vi "BH Druck  PACE Series Controller.vi"() -> ()   [LabVIEW 2022 SP3]
uses:
  <vilib>/Utility/error.llb/DialogType.ctl
  BH Druck PACE Series.lvclass
panel:
  out "Pressure":dbl format="%#.10g"
  out "+ve Source":dbl format="%#.10g"
  out "-ve Source":dbl format="%#.10g"
  in  "stop":bool
  out "Time to In Limits":string
  out "In Limits":bool
  out "Barometer":dbl format="%#.10g"
  in  "Enable Controller":bool
  in  "Slew Rate (0)":dbl
  in  "Slew Mode (Maximum)":string(combo)="max"
  in  "Overshoot (0: Not Allowed)":u16(ring)=1 items=["Not Allowed", "Allowed"]
  in  "Unit (mbar)":u16(ring) items=["mbar", "bar", "Pa", "hPa", "kPa", "mPa", "mmHg@0°C", "cmHg@0°C", "mHg@0°C", "inHg@0°C", "kg/cm2", "kg/m2", "mmH2O@4°C", "cmH2O@4°C", "mH2O@4°C", "mmH2O@20°C", "cmH2O@20°C", "mH2O@20°C", "torr", "atm", "psi", "lb/ft2", "inH2O@4°C", "inH2O@20°C", "inH2O@60°F", "ftH2O@4°C", "ftH2O@20°C", "ftH2O@60°F", "UserUnit1", "UserUnit2", "UserUnit3", "UserUnit4"]
  in  "Setpoint Value (0)":dbl
  out "Range":string
  out "-ve Full Scale":dbl
  out "+ve Full Scale":dbl
  in  "Channel (0: Channel A)":u16(ring) items=["Channel A", "Channel B"]
  in  "VISA resource name":refnum<visa-resource-name>
  # "(c)2010-2017 BH  Druck Ltd.  ALL RIGHTS RESERVED."
  # "Select port and channel"
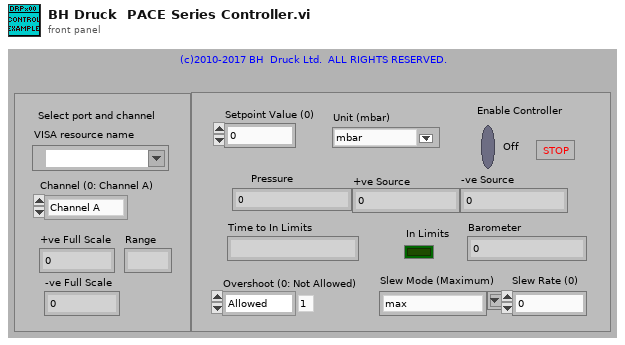
[diagram p1: front panel]
types:
  T1 = typedef "DialogType.ctl" = u16
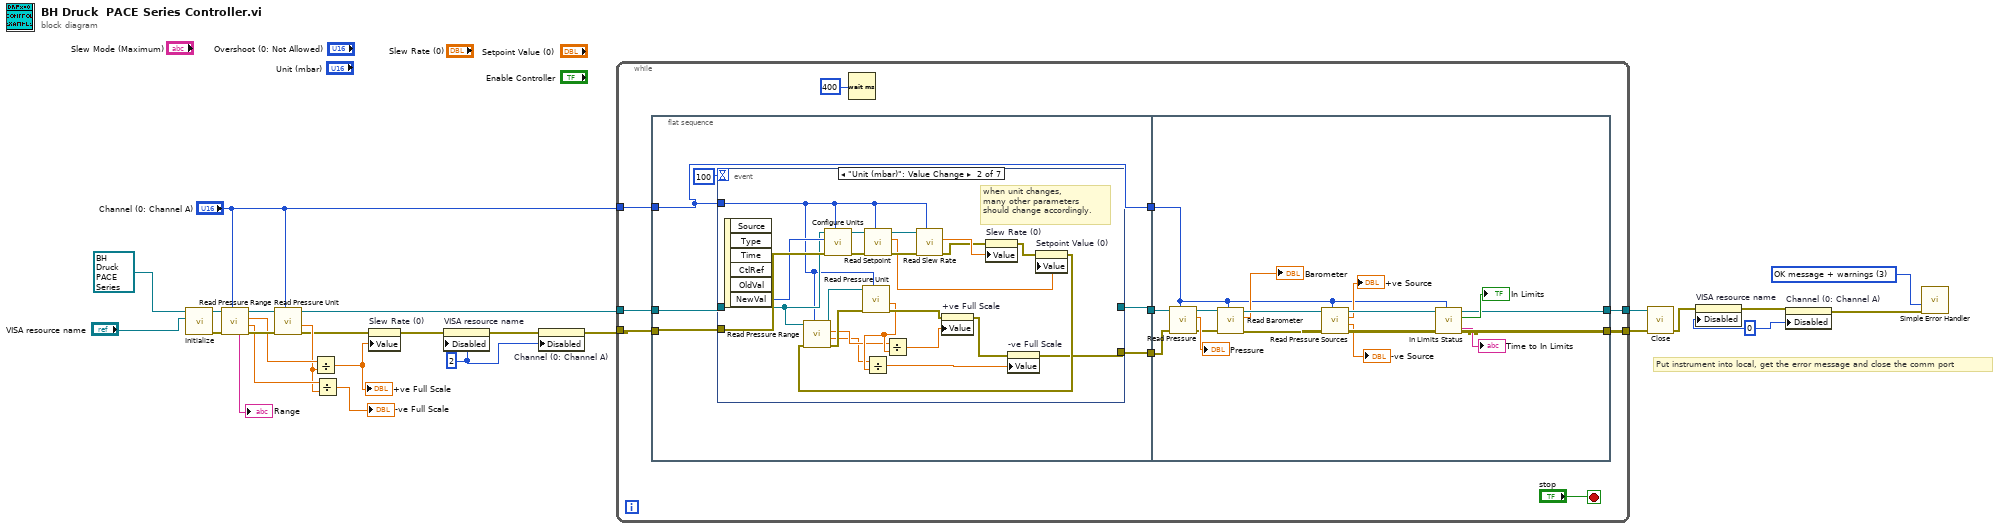
[diagram p0: block diagram]
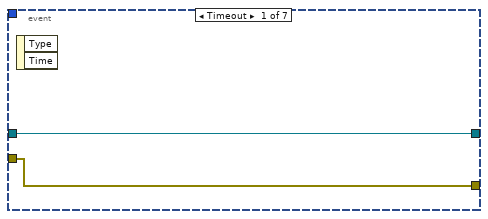
[diagram p2: hidden frame]
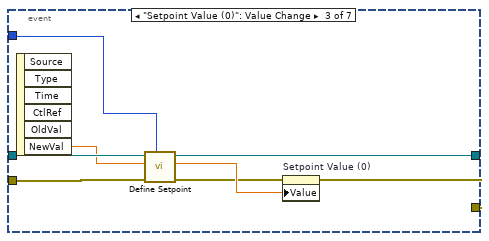
[diagram p3: hidden frame]
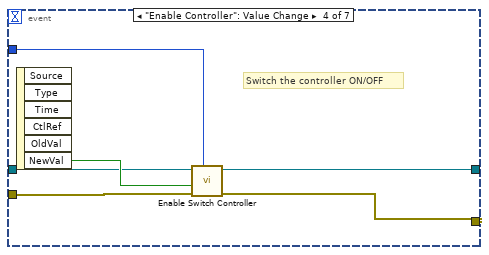
[diagram p4: hidden frame]
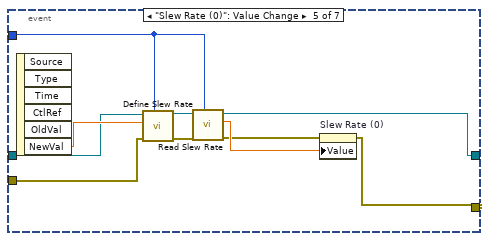
[diagram p5: hidden frame]
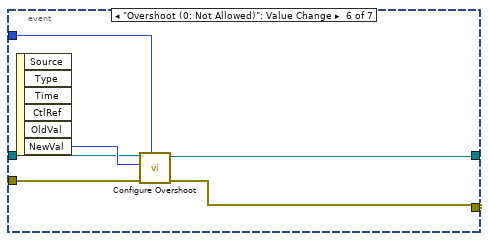
[diagram p6: hidden frame]
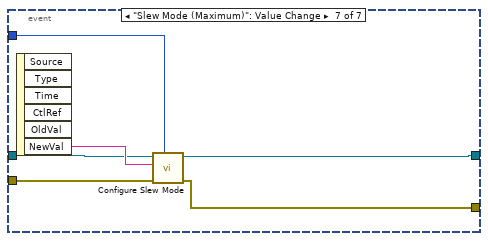
[diagram p7: hidden frame]
diagram:
  w2 = T1 3 items=["no dialog", "OK message", "continue or stop message", "OK message + warnings", "continue/stop + warnings"] ("type of dialog (OK msg:1)")
  w10 = u8 0 ("Disabled")
  w16 = u8 2 ("Disabled")
  # "Put instrument into local, get the error message and close the comm port"
  n1 = call-dynamic "Initialize.vi"("VISA resource name"="VISA resource name", "BH Druck PACE Series in"=refnum<class "BH Druck PACE Series.lvclass"> refnum) -> ("error out"=w4:errorcluster, "BH Druck PACE Series out"=w5:refnum<class "BH Druck PACE Series.lvclass">)  [unwired: 7 in]
  n2 = call-dynamic "Read Pressure Range.vi"("Channel (0: Channel A)"="Channel (0: Channel A)", "error in (no error)"=w4, "BH Druck PACE Series in"=w5) -> ("error out"=w23:errorcluster, "-FS Range/mbar"=w21:dbl, "+FS Range/mbar"=w22:dbl, "BH Druck PACE Series out"=w24:refnum<class "BH Druck PACE Series.lvclass">, "Range"=→"Range":string)  [unwired: 4 in]
  n3 = call-dynamic "Read Pressure Unit.vi"("Channel (0: Channel A)"="Channel (0: Channel A)", "error in (no error)"=w23, "BH Druck PACE Series in"=w24) -> ("error out"=w14:errorcluster, "Unit Convert"=w20:dbl, "BH Druck PACE Series out"=w7:refnum<class "BH Druck PACE Series.lvclass">)  [unwired: 5 in, 1 out]
  n4 = Divide(x=w22, y=w20) -> (x/y=w15:dbl)
  "+ve Full Scale" <- w15
  n5 = Divide(x=w21, y=w20) -> (x/y=→"-ve Full Scale":dbl)
  n6 = property on="Slew Rate (0)" class="DigNum (strict)"(error in=w14, "Value"=w15) -> (error out=w13:errorcluster)  [unwired: 1 in, 1 out]
  n7 = property on="VISA resource name" class="VISAName"(error in=w13, "Disabled"=w16) -> (error out=w17:errorcluster)  [unwired: 1 in, 1 out]
  n8 = property on="Channel (0: Channel A)" class="Ring (strict)"(error in=w17, "Disabled"=w16) -> (error out=w6:errorcluster)  [unwired: 1 in, 1 out]
  n9 = while {
    tunnel: w7 -> [w34]
    tunnel: w6 -> [w33]
    tunnel: "Channel (0: Channel A)" -> [w32]
    tunnel: [w31] -> w9
    tunnel: [w30] -> w8
    stop <- "stop" stop-if-true
    n10 = flat-sequence {
      tunnel: w34 -> [w40]
      tunnel: [w37] -> w29
      tunnel: w33 -> [w41]
      tunnel: w32 -> [w39]
      tunnel: [w39] -> w28
      tunnel: [w38] -> w27
      tunnel: w29 -> [w119]
      tunnel: w28 -> [w104]
      tunnel: [w107] -> w31
      tunnel: [w105] -> w30
      tunnel: w27 -> [w106]
      frame #0 {
        n11 = event shown="[1] \"Unit (mbar)\": Value Change" {
          selector: _ -> [_ _ _ _ _ _ _]
          dyn-events: _ -> [_ _ _ _ _ _ _]
          timeout: 100 -> [_ _ _ _ _ _ _]
          tunnel: w40 -> [w43 w51 w75 w80 w90 w95 w101]
          tunnel: w39 -> [_ w46 w72 w79 w87 w96 w102]
          tunnel: w41 -> [w44 w57 w73 w78 w89 w94 w100]
          tunnel: [w44 w45 w69 w77 w84 w93 w99] -> w38
          tunnel: [w43 _ w68 w76 w82 w92 w98] -> w37
          event Timeout {
            n12 = event-data() -> ()  [unwired: 1 in, 2 out]
          }
          event "Unit (mbar)": Value Change {
            # "when unit changes,\nmany other parameters\nshould change accordingly."
            n13 = event-data() -> ("NewVal"=w55:u16)  [unwired: 1 in, 5 out]
            n14 = call-dynamic "Configure Units.vi"("Channel (0: Channel A)"=w46, "error in (no error)"=w57, "Unit (mbar)"=w55, "BH Druck PACE Series in"=w51) -> ("error out"=w64:errorcluster, "BH Druck PACE Series out"=w65:refnum<class "BH Druck PACE Series.lvclass">)  [unwired: 6 in]
            n15 = call-dynamic "Read Setpoint.vi"("Channel (0: Channel A)"=w46, "error in (no error)"=w64, "BH Druck PACE Series in"=w65) -> ("error out"=w67:errorcluster, "Setpoint"=w54:dbl, "BH Druck PACE Series out"=w66:refnum<class "BH Druck PACE Series.lvclass">)  [unwired: 6 in]
            n16 = call-dynamic "Read Slew Rate.vi"("Channel (0: Channel A)"=w46, "error in (no error)"=w67, "BH Druck PACE Series in"=w66) -> ("error out"=w56:errorcluster, "Slew Rate Measurement"=w59:dbl)  [unwired: 6 in, 1 out]
            n17 = property on="Slew Rate (0)" class="DigNum (strict)"(error in=w56, "Value"=w59) -> (error out=w53:errorcluster)  [unwired: 1 in, 1 out]
            n18 = property on="Setpoint Value (0)" class="DigNum (strict)"(error in=w53, "Value"=w54) -> (error out=w52:errorcluster)  [unwired: 1 in, 1 out]
            n19 = call-dynamic "Read Pressure Range.vi"("Channel (0: Channel A)"=w46, "error in (no error)"=w52, "BH Druck PACE Series in"=w51) -> ("error out"=w50:errorcluster, "-FS Range/mbar"=w48:dbl, "+FS Range/mbar"=w49:dbl, "BH Druck PACE Series out"=w47:refnum<class "BH Druck PACE Series.lvclass">)  [unwired: 4 in, 1 out]
            n20 = call-dynamic "Read Pressure Unit.vi"("Channel (0: Channel A)"=w46, "error in (no error)"=w50, "BH Druck PACE Series in"=w47) -> ("error out"=w62:errorcluster, "Unit Convert"=w58:dbl)  [unwired: 5 in, 2 out]
            n21 = Divide(x=w48, y=w58) -> (x/y=w61:dbl)
            n22 = Divide(x=w49, y=w58) -> (x/y=w63:dbl)
            n23 = property on="+ve Full Scale" class="DigNum (strict)"(error in=w62, "Value"=w63) -> (error out=w60:errorcluster)  [unwired: 1 in, 1 out]
            n24 = property on="-ve Full Scale" class="DigNum (strict)"(error in=w60, "Value"=w61) -> (error out=w45:errorcluster)  [unwired: 1 in, 1 out]
          }
          event "Setpoint Value (0)": Value Change {
            n25 = event-data() -> ("NewVal"=w74:dbl)  [unwired: 1 in, 5 out]
            n26 = call-dynamic "Define Setpoint.vi"("Channel (0: Channel A)"=w72, "error in (no error)"=w73, "Setpoint Value"=w74, "BH Druck PACE Series in"=w75) -> ("error out"=w70:errorcluster, "Setpoint Issued"=w71:dbl, "BH Druck PACE Series out"=w68:refnum<class "BH Druck PACE Series.lvclass">)  [unwired: 5 in]
            n27 = property on="Setpoint Value (0)" class="DigNum (strict)"(error in=w70, "Value"=w71) -> (error out=w69:errorcluster)  [unwired: 1 in, 1 out]
          }
          event "Enable Controller": Value Change {
            # "Switch the controller ON/OFF"
            n28 = event-data() -> ("NewVal"=w81:bool)  [unwired: 1 in, 5 out]
            n29 = call-dynamic "Enable Switch Controller.vi"("Channel (0: Channel A)"=w79, "error in (no error)"=w78, "Enable Controller (Off)"=w81, "BH Druck PACE Series in"=w80) -> ("error out"=w77:errorcluster, "BH Druck PACE Series out"=w76:refnum<class "BH Druck PACE Series.lvclass">)  [unwired: 6 in]
          }
          event "Slew Rate (0)": Value Change {
            n30 = event-data() -> ("NewVal"=w91:dbl)  [unwired: 1 in, 5 out]
            n31 = call-dynamic "Define Slew Rate.vi"("Channel (0: Channel A)"=w87, "error in (no error)"=w89, "Slew Rate (100)"=w91, "BH Druck PACE Series in"=w90) -> ("error out"=w86:errorcluster, "BH Druck PACE Series out"=w88:refnum<class "BH Druck PACE Series.lvclass">)  [unwired: 5 in, 1 out]
            n32 = call-dynamic "Read Slew Rate.vi"("Channel (0: Channel A)"=w87, "error in (no error)"=w86, "BH Druck PACE Series in"=w88) -> ("error out"=w83:errorcluster, "Slew Rate Measurement"=w85:dbl, "BH Druck PACE Series out"=w82:refnum<class "BH Druck PACE Series.lvclass">)  [unwired: 6 in]
            n33 = property on="Slew Rate (0)" class="DigNum (strict)"(error in=w83, "Value"=w85) -> (error out=w84:errorcluster)  [unwired: 1 in, 1 out]
          }
          event "Overshoot (0: Not Allowed)": Value Change {
            n34 = event-data() -> ("NewVal"=w97:u16)  [unwired: 1 in, 5 out]
            n35 = call-dynamic "Configure Overshoot.vi"("Channel (0: Channel A)"=w96, "error in (no error)"=w94, "Overshoot (1: Allowed)"=w97, "BH Druck PACE Series in"=w95) -> ("error out"=w93:errorcluster, "BH Druck PACE Series out"=w92:refnum<class "BH Druck PACE Series.lvclass">)  [unwired: 6 in]
          }
          event "Slew Mode (Maximum)": Value Change {
            n36 = event-data() -> ("NewVal"=w103:string)  [unwired: 1 in, 5 out]
            n37 = call-dynamic "Configure Slew Mode.vi"("Channel (0: Channel A)"=w102, "error in (no error)"=w100, "Slew Mode (Maximum)"=w103, "BH Druck PACE Series in"=w101) -> ("error out"=w99:errorcluster, "BH Druck PACE Series out"=w98:refnum<class "BH Druck PACE Series.lvclass">)  [unwired: 6 in]
          }
        }
      }
      frame #1 {
        n38 = call-dynamic "Read Pressure.vi"("Channel (0: Channel A)"=w104, "error in (no error)"=w106, "BH Druck PACE Series in"=w119) -> ("error out"=w117:errorcluster, "Measured Pressure"=→"Pressure":dbl, "BH Druck PACE Series out"=w114:refnum<class "BH Druck PACE Series.lvclass">)  [unwired: 6 in]
        n39 = call-dynamic "Read Barometer.vi"("Channel (0: Channel A)"=w104, "error in (no error)"=w117, "BH Druck PACE Series in"=w114) -> ("error out"=w116:errorcluster, "Barometer"=→"Barometer":dbl, "BH Druck PACE Series out"=w113:refnum<class "BH Druck PACE Series.lvclass">)  [unwired: 6 in]
        n40 = call-dynamic "Read Pressure Sources.vi"("Channel (0: Channel A)"=w104, "error in (no error)"=w116, "BH Druck PACE Series in"=w113) -> ("error out"=w115:errorcluster, "Vacuum Sensor -ve Source"=→"-ve Source":dbl, "Pressure Sensor  +ve Source"=→"+ve Source":dbl, "BH Druck PACE Series out"=w112:refnum<class "BH Druck PACE Series.lvclass">)  [unwired: 5 in]
        n41 = call-dynamic "In Limits Status.vi"("Channel (0: Channel A)"=w104, "error in (no error)"=w115, "BH Druck PACE Series in"=w112) -> ("error out"=w105:errorcluster, "In Limits"=→"In Limits":bool, "BH Druck PACE Series out"=w107:refnum<class "BH Druck PACE Series.lvclass">, "Time to In Limits"=→"Time to In Limits":string)  [unwired: 4 in, 1 out]
      }
    }
    n42 = Wait (ms)(milliseconds to wait=u32 400) -> ()  [unwired: 1 out]
  }
  n43 = call "Close.vi"("error in (no error)"=w8, "BH Druck PACE Series in"=w9) -> ("error out"=w12:errorcluster)  [unwired: 8 in, 1 out]
  n44 = property on="VISA resource name" class="VISAName"(error in=w12, "Disabled"=w10) -> (error out=w11:errorcluster)  [unwired: 1 in, 1 out]
  n45 = property on="Channel (0: Channel A)" class="Ring (strict)"(error in=w11, "Disabled"=w10) -> (error out=w3:errorcluster)  [unwired: 1 in, 1 out]
  n46 = call <vilib>:"Simple Error Handler.vi"("type of dialog (OK msg:1)"=w2, "error in (no error)"=w3) -> ()  [unwired: 3 in, 5 out]
